vi "final.vi"() -> ()   [LabVIEW 2012]
uses:
  Global 1.vi
panel:
  in  "File Path:\nManually Type the path, unless the file already exists.":path
  in  "STOP":bool
  out "Frequency":string
  out "Phase":string
  out "VX":string
  in  "Time Delay (sec)":u32
  in  "error in (no error) 3":errorcluster
  in  "Set Increment":string
  in  "Set Final Frequency":string
  in  "Set Initial Frequency":string
  out "VR":string
  out "VY":string
  in  "Set GPIB":refnum<visa-resource-name>
  out "File Path":path
  in  "File Comments":string
  in  "File Name":string caption="Beginning Text"
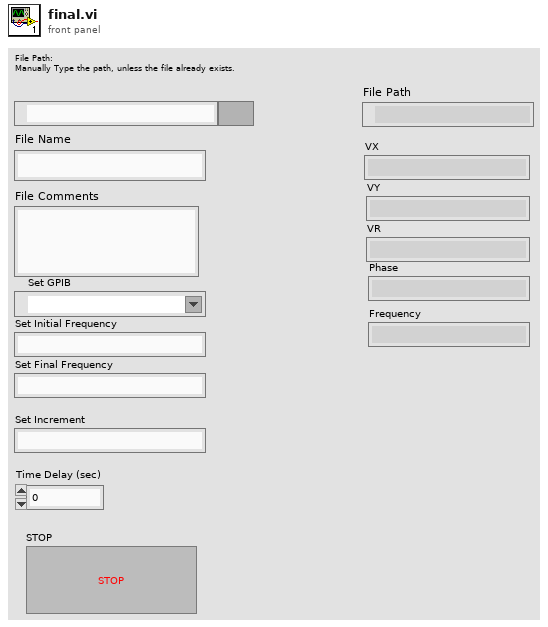
[diagram p1: front panel]
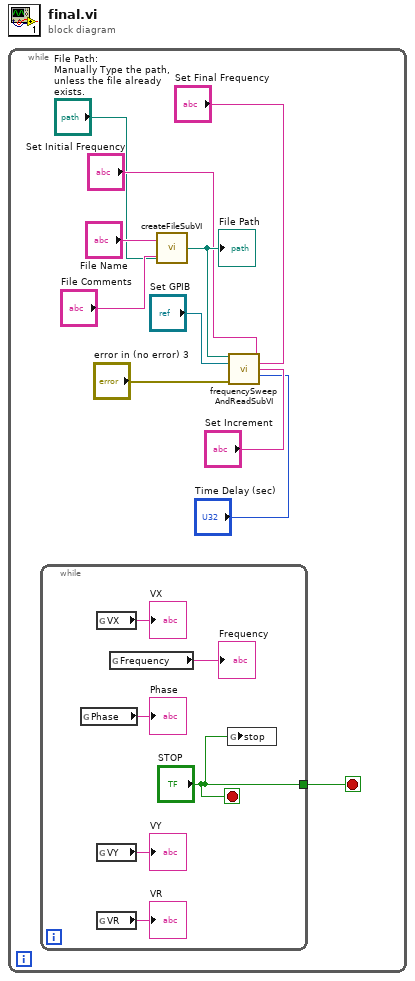
[diagram p0: block diagram]
diagram:
  n1 = while {
    stop <- w2 stop-if-true
    n2 = while {
      tunnel: ["STOP"] -> w2
      stop <- "STOP" stop-if-true
      n3 = global read "Global 1.vi" "Phase"() -> (→"Phase":string)
      n4 = global read "Global 1.vi" "VX"() -> (→"VX":string)
      n5 = global read "Global 1.vi" "VY"() -> (→"VY":string)
      n6 = global read "Global 1.vi" "VR"() -> (→"VR":string)
      n7 = global read "Global 1.vi" "Frequency"() -> (→"Frequency":string)
      n8 = global write "Global 1.vi" "stop"("STOP") -> ()
    }
    n9 = call "createFileSubVI.vi"("File Name"="File Name", "File Comments"="File Comments", "Path For File,\nManually Type the path, unless the file already exists."="File Path:\nManually Type the path, unless the file already exists.") -> ("File Path"=w9:path)  [unwired: 1 out]
    "File Path" <- w9
    n10 = call "frequencySweepAndReadSubVI.vi"("file (use dialog)"=w9, "Set Initial Frequency"="Set Initial Frequency", "Set GPIB"="Set GPIB", "Set Final Frequency"="Set Final Frequency", "Set Increment"="Set Increment", "Time Delay (sec)"="Time Delay (sec)", "error in (no error) 3"="error in (no error) 3") -> ()  [unwired: 4 in, 5 out]
  }
